vi "VI_UsingTypeDef.vi"(11 "Cluster In":T1) -> (3 "Cluster Out":T1)   [LabVIEW 2012]
uses:
  LabVIEWControlStrictTypeDef.ctl
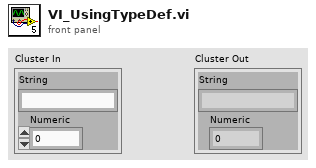
[diagram p1: front panel]
types:
  T1 = typedef "LabVIEWControlStrictTypeDef.ctl" = cluster{"String":string, "Numeric":dbl}
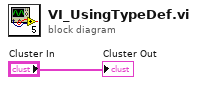
[diagram p0: block diagram]
diagram:
  "Cluster Out" <- "Cluster In"
